vi "校准.vi"(1 "字符串":string="@01????????P") -> (0 "连接的字符串":string)   [LabVIEW 2015]
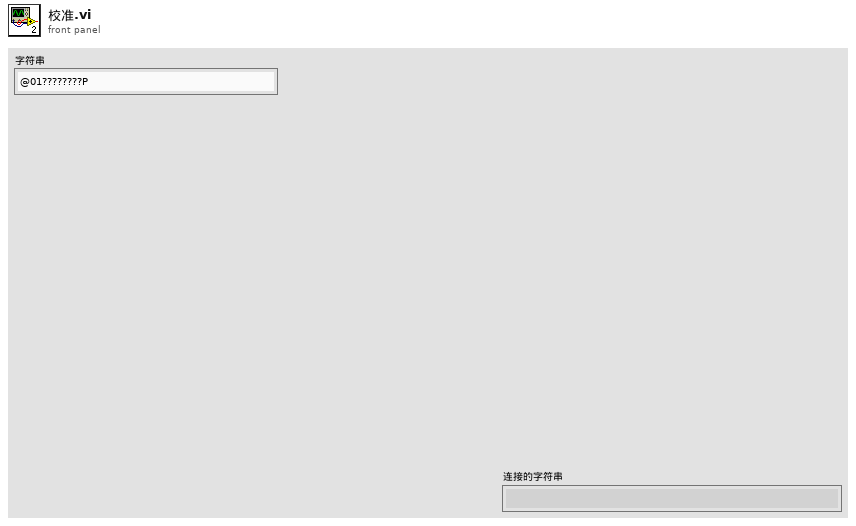
[diagram p1: front panel]
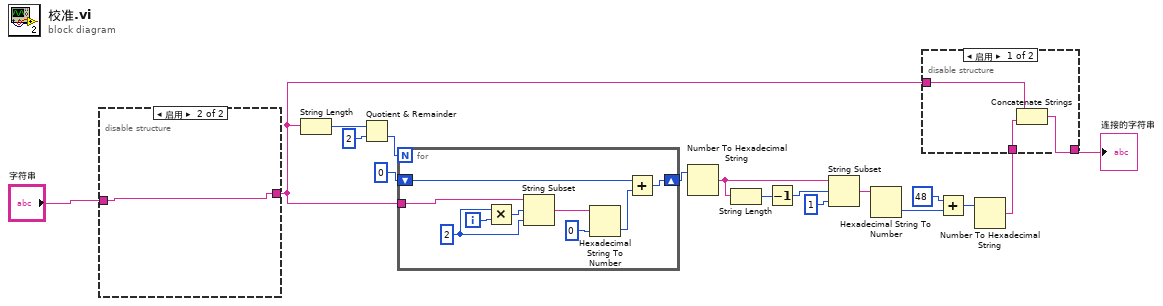
[diagram p0: block diagram]
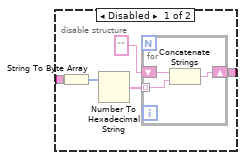
[diagram p2: hidden frame]
diagram:
  n1 = disable-structure shown="启用" {
    disable-tunnel: "字符串" -> [w22 w26]
    disable-tunnel: [w18 w26] -> w3
    frame Disabled {
      n2 = String To Byte Array(string=w22) -> (unsigned byte array=w20:u8[])
      n3 = Number To Hexadecimal String(2:w20) -> (0:w19:string[])  [unwired: 1 in]
      n4 = for {
        tunnel: w19 -> [w24] mode=indexing
        shift-right: [w23] -> w18
        shift-left: "" ("字符串") -> [w25]
        n5 = Concatenate Strings(w25, w24) -> (w23:string)
      }
    }
    frame Enabled {
    }
  }
  n6 = String Length(string=w3) -> (length=w16:i32)
  n7 = Quotient & Remainder(x=w16, y=2) -> (floor(x/y)=w14:i32)  [unwired: 1 out]
  n8 = for {
    N: w14 -> [_]
    shift-right: [w30] -> w12
    shift-left: u64 0 -> [w32]
    tunnel: w3 -> [w31]
    i -> [w35]
    w33 = 2
    n9 = Multiply(x=w33, y=w35) -> (x*y=w34:i32)
    n10 = String Subset(string=w31, offset (0)=w34, length (rest)=w33) -> (substring=w29:string)
    n11 = Hexadecimal String To Number(string=w29, default (0uL)=u64 0 ("默认(0 U32)")) -> (number=w28:u64)  [unwired: 1 in, 1 out]
    n12 = Add(x=w32, y=w28) -> (x+y=w30:u64)
  }
  n13 = Number To Hexadecimal String(2:w12) -> (0:w11:string)  [unwired: 1 in]
  n14 = String Length(string=w11) -> (length=w10:i32)
  n15 = Decrement(x=w10) -> (x-1=w9:i32)
  n16 = String Subset(string=w11, offset (0)=w9, length (rest)=1 ("长度（剩余）")) -> (substring=w7:string)
  n17 = Hexadecimal String To Number(string=w7) -> (number=w5:u32)  [unwired: 2 in, 1 out]
  n18 = Add(x=u8 48, y=w5) -> (x+y=w4:u32)
  n19 = Number To Hexadecimal String(2:w4) -> (0:w2:string)  [unwired: 1 in]
  n20 = disable-structure shown="启用" {
    disable-tunnel: w3 -> [w38 _]
    disable-tunnel: w2 -> [w37 w39]
    disable-tunnel: [w36 w39] -> w1
    frame Enabled {
      n21 = Concatenate Strings(w38, w37) -> (w36:string)
    }
    frame Disabled {
    }
  }
  "连接的字符串" <- w1
